vi "test_AK TCP Write.vi"(8 "error in (no error)":errorcluster, 11 "TestCase in":refnum<class "Ethernet Protocol Tests.lvclass">) -> (0 "error out":errorcluster, 3 "TestCase out":refnum<class "Ethernet Protocol Tests.lvclass">)   [LabVIEW 2019, in "Ethernet Protocol Tests.lvclass"]
uses:
  Ethernet Protocol Tests.lvclass
  Listener/Listener.lvclass
  Listener/ListenerClassControls/Operation.ctl
  AK TCP/AK TCP.lvclass
  D:/GitRepository/niveristand-instrument-addon-classes/Source/Protocols/TCP/TCP.lvclass
  D:/GitRepository/niveristand-instrument-addon-classes/Source/Protocols/Protocol Parent/Protocol Parent.lvclass
  TCP/TCP.lvclass/TCP.ctl
  Constants.vi
  <vilib>/addons/_JKI Toolkits/VI Tester/TestCase.llb/TestCase.lvclass
  TCP/TCP.lvclass
  C:/Program Files (x86)/National Instruments/LabVIEW 2019/vi.lib/addons/_JKI Toolkits/VI Tester/TestCase.llb/TestCase.lvclass
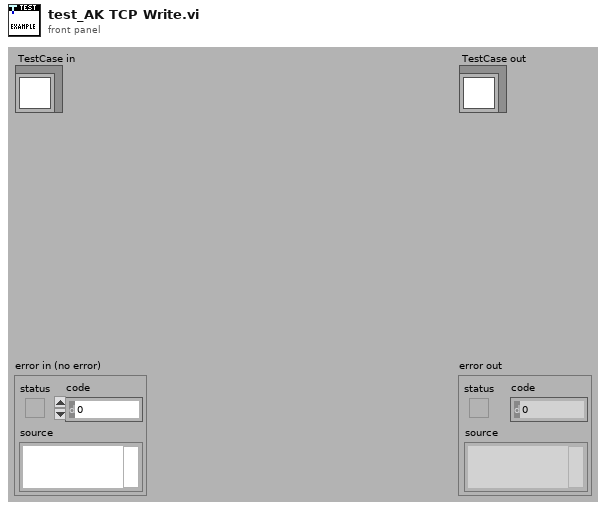
[diagram p1: front panel]
types:
  T1 = typedef "Listener.lvclass/Operation.ctl" = enum16{"Read", "Write"}
  T2 = typedef "Listener.lvclass/AK TCP Data Structure.ctl" = cluster{"TCP|IP connection ID":refnum<k5>, "IP Address":string, "Port":u16, "Data":string, "Current Command Code":string}
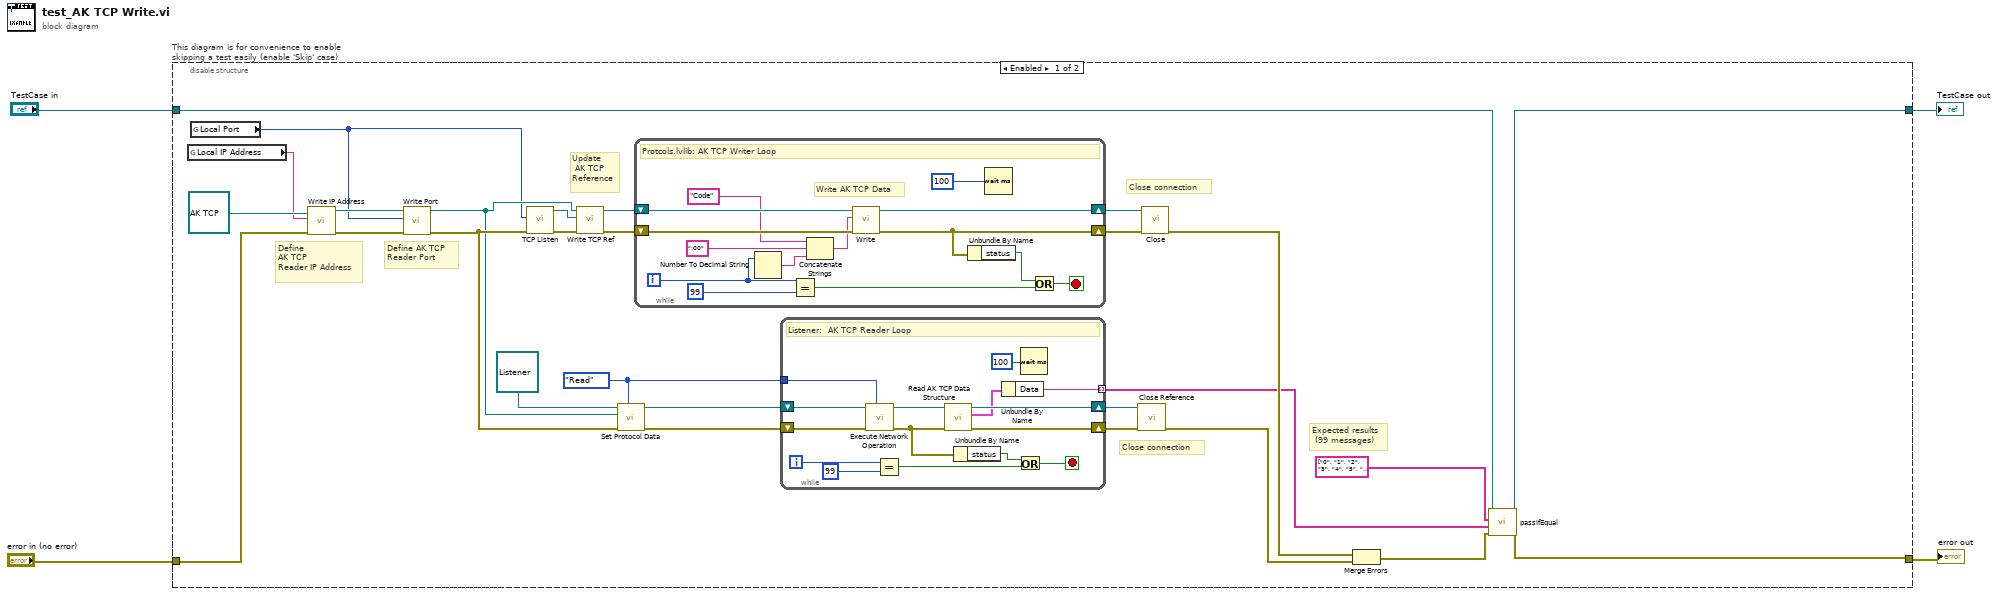
[diagram p0: block diagram]
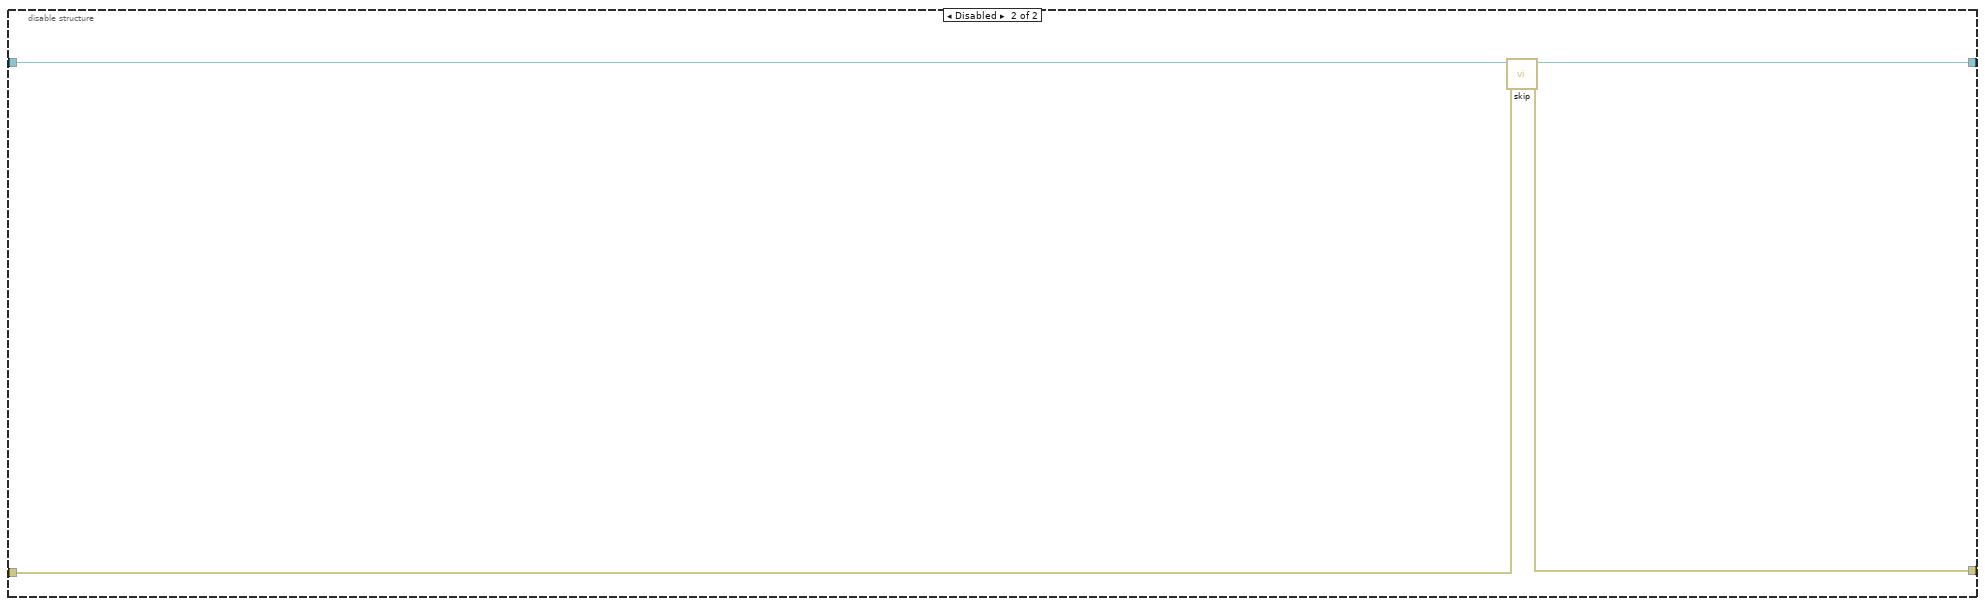
[diagram p2: hidden frame]
diagram:
  n1 = disable-structure "This diagram is for convenience to enable skipping a test easily (enable 'Skip' case)" shown="Enabled" {
    disable-tunnel: "TestCase in" -> [w32 w65]
    disable-tunnel: [w31 w63] -> w1
    disable-tunnel: [w30 w64] -> w3
    disable-tunnel: "error in (no error)" -> [w27 w62]
    frame Enabled {
      w16 = Operation."Read" ("Operation")
      # "Close connection"
      # "Close connection"
      # "Update\n AK TCP \nReference"
      # "Expected results\n (99 messages)"
      # "Define AK TCP \nReader Port"
      # "Define \nAK TCP \nReader IP Address"
      n2 = global read "Constants.vi" "Local IP Address"() -> (w6:string)
      n3 = global read "Constants.vi" "Local Port"() -> (w5:u16)
      n4 = call "Write IP Address.vi"("error in (no error)"=w27, "IP Address"=w6, "Ethernet in"=refnum<class "AK TCP.lvclass"> refnum ("Protocols.lvlib:AK TCP.lvclass")) -> ("error out"=w28:errorcluster, "Ethernet out"=w29:refnum<class "AK TCP.lvclass">)  [unwired: 7 in]
      n5 = call "Write Port.vi"("error in (no error)"=w28, "Port"=w5, "Ethernet in"=w29) -> ("error out"=w22:errorcluster, "Ethernet out"=w18:refnum<class "AK TCP.lvclass">)  [unwired: 7 in]
      n6 = call <vilib>:"TCP Listen.vi"("error in (no error)"=w22, "port"=w5) -> ("error out"=w21:errorcluster, "connection ID"=w17:refnum<k5>)  [unwired: 5 in, 3 out]
      n7 = call "Write TCP Ref.vi"("error in (no error)"=w21, "TCP Ref"=w17, "Ethernet in"=w18) -> ("error out"=w20:errorcluster, "Ethernet out"=w19:refnum<class "AK TCP.lvclass">)  [unwired: 7 in]
      n8 = call "Set Protocol Data.vi"("Operation"=w16, "error in (no error)"=w22, "Protocols.lvlib:Protocol Parent.lvclass"=w18, "Listener In.lvclass"=refnum<class "Listener.lvclass"> refnum ("Listener.lvclass")) -> ("error out"=w23:errorcluster, "Listener Out.lvclass"=w24:refnum<class "Listener.lvclass">)  [unwired: 6 in]
      n9 = while {
        shift-right: [w55] -> w12
        shift-left: w20 -> [w53]
        shift-right: [w56] -> w11
        shift-left: w19 -> [w57]
        i -> [w52]
        stop <- w60 stop-if-true
        # "Write AK TCP Data"
        # "Protcols.lvlib: AK TCP Writer Loop"
        n10 = Number To Decimal String(number=w52) -> (decimal integer string=w51:string)  [unwired: 1 in]
        n11 = Equal?(x=w52, y=99 ("x")) -> (x = y?=w61:bool)
        n12 = Concatenate Strings("Code" ("string"), ":00" ("string"), w51) -> (w49:string)
        n13 = call-dynamic "Write.vi"("error in (no error)"=w53, "String"=w49, "AK TCP in"=w57) -> ("error out"=w55:errorcluster, "AK TCP out"=w56:refnum<class "AK TCP.lvclass">)  [unwired: 7 in]
        n14 = Unbundle By Name(w55) -> ("status"=w54:bool)
        n15 = Wait (ms)(milliseconds to wait=u32 100) -> ()  [unwired: 1 out]
        n16 = Or(x=w54, y=w61) -> (x .or. y?=w60:bool)
      }
      n17 = while {
        shift-right: [w35] -> w14
        shift-left: w23 -> [w47]
        shift-right: [w34] -> w15
        shift-left: w24 -> [w46]
        tunnel: w16 -> [w41]
        tunnel: [w40] -> w9 mode=indexing
        i -> [w39]
        stop <- w44 stop-if-true
        # "Listener:  AK TCP Reader Loop"
        n18 = call "Execute Network Operation.vi"("Operation"=w41, "error in (no error)"=w47, "Listener In.lvclass"=w46) -> ("error out"=w37:errorcluster, "Listener Out.lvclass"=w36:refnum<class "Listener.lvclass">)  [unwired: 7 in]
        n19 = Equal?(x=w39, y=99 ("x")) -> (x = y?=w43:bool)
        n20 = call-dynamic "Read AK TCP Data Structure.vi"("error in (no error)"=w37, "Listener in"=w36) -> ("error out"=w35:errorcluster, "TCP|IP Data Structure"=w33:T2, "Listener out"=w34:refnum<class "Listener.lvclass">)  [unwired: 7 in]
        n21 = Unbundle By Name(w37) -> ("status"=w45:bool)
        n22 = Unbundle By Name(w33) -> ("Data"=w40:string)
        n23 = Or(x=w45, y=w43) -> (x .or. y?=w44:bool)
        n24 = Wait (ms)(milliseconds to wait=u32 100) -> ()  [unwired: 1 out]
      }
      n25 = call "Close Reference.vi"("error in (no error)"=w14, "Listener In.lvclass"=w15) -> ("error out"=w13:errorcluster)  [unwired: 9 in]
      n26 = call-dynamic "Close.vi"("error in (no error)"=w12, "Ethernet in"=w11) -> ("error out"=w10:errorcluster)  [unwired: 8 in, 1 out]
      n27 = Merge Errors(w10, w13) -> (w26:errorcluster)
      n28 = call-dynamic "passIfEqual.vi"("error in (no error)"=w26, "y"=w9, "x"=string[] ["0", "1", "2", "3", "4", "5", "6", "7", "8", "9", "10", "11", "12", "13", "14", "15", "16", "17", "18", "19", "20", "21", "22", "23", "24", "25", "26", "27", "28", "29", "30", "31", "32", "33", "34", "35", "36", "37", "38", "39", "40", "41", "42", "43", "44", "45", "46", "47", "48", "49", "50", "51", "52", "53", "54", "55", "56", "57", "58", "59", "60", "61", "62", "63", "64", "65", "66", "67", "68", "69", "70", "71", "72", "73", "74", "75", "76", "77", "78", "79", "80", "81", "82", "83", "84", "85", "86", "87", "88", "89", "90", "91", "92", "93", "94", "95", "96", "97", "98", "99"] ("Array"), "TestCase in"=w32) -> ("error out"=w30:errorcluster, "TestCase out"=w31:refnum<class "Ethernet Protocol Tests.lvclass">)  [unwired: 6 in]
    }
    frame Disabled {
      # "skip test result while test is under development"
      n29 = call <vilib>:"skip.vi"("error in (no error)"=w62, "TestCase in"=w65) -> ("error out"=w64:errorcluster, "TestCase out"=w63:refnum<class "Ethernet Protocol Tests.lvclass">)  [unwired: 8 in]
    }
  }
  "error out" <- w3
  "TestCase out" <- w1
